vi "Set (subVi).vi"(0 "Exchange.lvclass":refnum<class "Exchange.lvclass">, 1 "endpoint":string, 2 "Channel in":refnum<class "Channel.lvclass">, 3 "error in (no error)":errorcluster, 4 "lockout_key":string, 6 "value":string, 8 "timeout":dbl=10.0 format="%#_13g") -> (5 "Array - String":string[](array[string]), 7 "timeout?":bool=TRUE, 9 "error out":errorcluster)   [LabVIEW 2016]
uses:
  <vilib>/Distrio/LabbitMQ/Exchange/Exchange.lvclass
  <vilib>/Distrio/LabbitMQ/Channel/Channel.lvclass
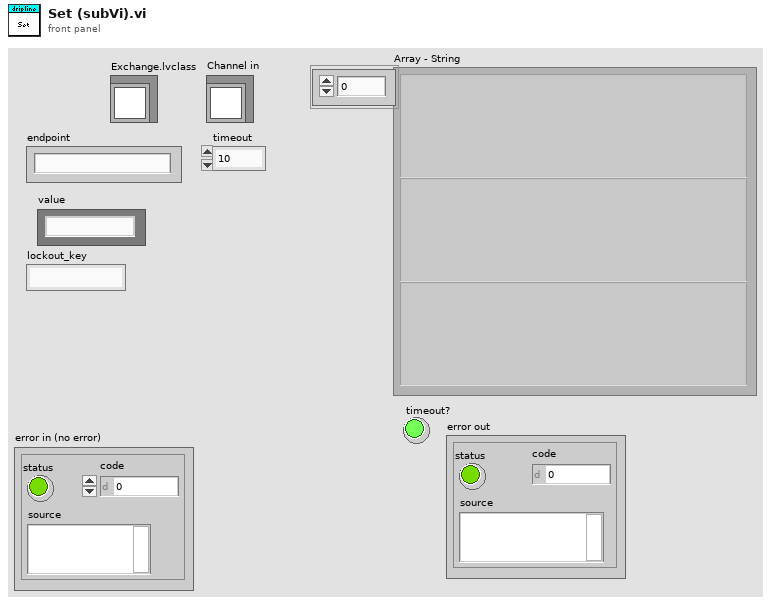
[diagram p1: front panel]
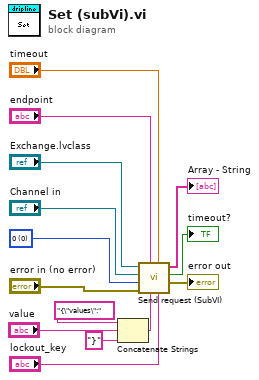
[diagram p0: block diagram]
diagram:
  w12 = 0 items=["0"=0, "1"=1, "6"=6, "7"=7, "8"=8, "9"=9] ("msgop")
  n1 = Concatenate Strings("{\"values\":" ("request content"), "value", "}" ("string")) -> (w3:string)
  n2 = call "Send request (SubVI).vi"("lockout_key"="lockout_key", "timeout"="timeout", "request content"=w3, "target"="endpoint", "error in (no error)"="error in (no error)", "msgop"=w12, "Channel in"="Channel in", "Exchange.lvclass"="Exchange.lvclass") -> ("error out"=→"error out":errorcluster, "timeout?"=→"timeout?":bool, "Array - String"=→"Array - String":string[])  [unwired: 1 in]
